vi "Init.vi"(8 "error in (no error)":errorcluster, 11 "PDE":refnum<class "NI_PDE.lvclass">) -> (0 "error out":errorcluster, 3 "initialized PDE":refnum<class "NI_PDE.lvclass">)   [LabVIEW 2020, in "NI_PDE.lvlib" / "NI_PDE.lvclass"]
uses:
  <vilib>/gmath/pde.llb/PDEClass/NI_PDE.lvclass
  <vilib>/gmath/pde.llb/PDEClass/Class Type.ctl
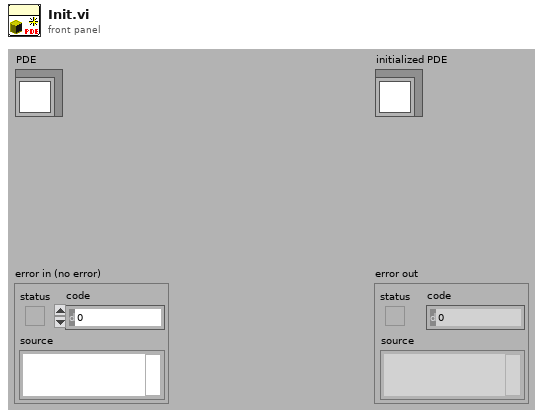
[diagram p1: front panel]
types:
  T1 = typedef "NI_PDE.lvlib/NI_PDE.lvclass/Class Type.ctl" = i32
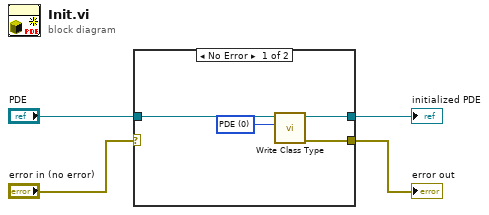
[diagram p0: block diagram]
diagram:
  n1 = case shown="No Error" "error in (no error)" {
    selector: "error in (no error)" -> [_ w10]
    tunnel: "PDE" -> [w7 w9]
    tunnel: [w6 w9] -> w3
    tunnel: [w5 w10] -> w2
    frame No Error {
      w8 = T1 0 items=["PDE"=0, "PDE_2ndOrder_ConstPara"=100, "PDE_Helmholtz_2D"=112, "PDE_Heat_1D"=121, "PDE_Heat_2D"=122, "PDE_Wave_1D"=131, "PDE_Wave_2D"=132] ("PDE class type")
      n2 = call-dynamic "Write Class Type.vi"("PDE class type"=w8, "PDE.lvclass in"=w7) -> ("error out"=w5:errorcluster, "PDE.lvclass out"=w6:refnum<class "NI_PDE.lvclass">)  [unwired: 1 in, 7 out]
    }
    frame Error {
    }
  }
  "initialized PDE" <- w3
  "error out" <- w2
